vi "On Compile - Cyclic Tx - Get Disable Channels Refs.vi"(8 "error in (no error)":errorcluster, 10 "Channel Data [] In":T1[](array[typedef]) {"Labels Settings"."Label Timestamp Channel Data Reference" format="%.0x"; "Labels Settings"."Label Disable/Trigger Channel Reference" format="%.0x"; "Labels Settings"."Word"."Param Setting"."Item Refs" format="%.0x"; "Labels Settings"."Word"."Param Setting"."Num Bits" min=1 max=32; "Labels Settings"."Word"."Param Setting"."Start Bit" min=8 max=31; "Labels Settings"."Label" format="%.0o"}) -> (0 "error out":errorcluster, 3 "Async Status Channels Refs":T13 {"VS Refs" format="%.0x"})   [LabVIEW 2019, in "Ballard Arinc-429 System Explorer.lvlib"]
uses:
  Ballard Arinc-429 System Explorer.lvlib
  <vilib>/NI VeriStand/Custom Device API/Custom Device Item Ref.ctl
  Shared/Controls and Global/RT HW Channel.ctl
  Shared/Controls and Global/RT Label Settings.ctl
  Shared/Controls and Global/Label.ctl
  Shared/Controls and Global/transferPeriod.ctl
  Shared/Controls and Global/RT Word Settings.ctl
  Shared/Controls and Global/RT Param Setting.ctl
  Shared/Controls and Global/Start Bit.ctl
  Shared/Controls and Global/Number of Bits.ctl
  <vilib>/NI VeriStand/Custom Device API/Block Data Reference.ctl
  <vilib>/NI VeriStand/Custom Device API/Data Reference.ctl
  Shared/Controls and Global/TransferType.ctl
  <vilib>/NI VeriStand/Custom Device API/Custom Device API.lvlib
  Shared/Ballard Arinc-429 Shared.lvlib
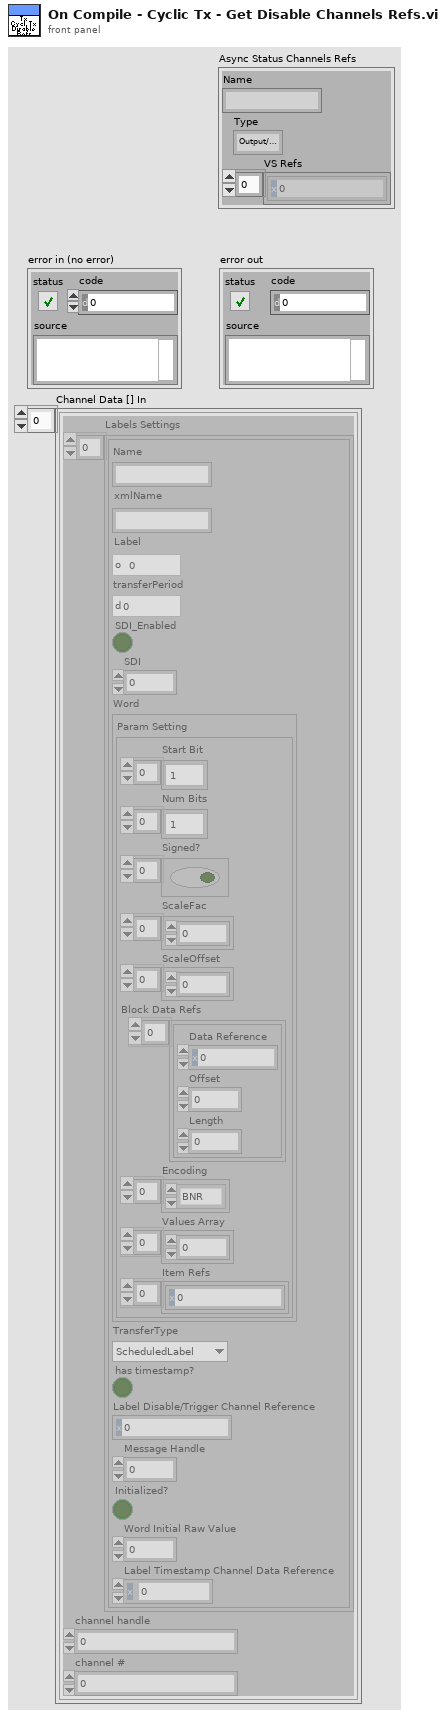
[diagram p1: front panel]
types:
  T1 = typedef "Ballard Arinc-429 Shared.lvlib/RT HW Channel.ctl" = cluster{"Labels Settings":T2[], "channel handle":u64, "channel #":u16}
  T2 = typedef "Ballard Arinc-429 Shared.lvlib/RT Label Settings.ctl" = cluster{"Name":string, "xmlName":string, "Label":T3, "transferPeriod":T4, "SDI_Enabled":bool, "SDI":u8, "Word":T5, "TransferType":T12, "has timestamp?":bool, "Label Disable/Trigger Channel Reference":T11, "Message Handle":u64, "Initialized?":bool, "Word Initial Raw Value":u32, "Label Timestamp Channel Data Reference":T10}
  T3 = typedef "Ballard Arinc-429 Shared.lvlib/Label.ctl" = u8
  T4 = typedef "Ballard Arinc-429 Shared.lvlib/transferPeriod.ctl" = u32
  T5 = typedef "Ballard Arinc-429 Shared.lvlib/RT Word Settings.ctl" = cluster{"Param Setting":T6}
  T6 = typedef "Ballard Arinc-429 Shared.lvlib/RT Param Setting.ctl" = cluster{"Start Bit":T7[], "Num Bits":T8[], "Signed?":bool[], "ScaleFac":dbl[], "ScaleOffset":dbl[], "Block Data Refs":T9[], "Encoding":enum16{"BNR", "BCD", "Discrete"}[], "Values Array":dbl[], "Item Refs":T11[]}
  T7 = typedef "Ballard Arinc-429 Shared.lvlib/Start Bit.ctl" = i32
  T8 = typedef "Ballard Arinc-429 Shared.lvlib/Number of Bits.ctl" = i32
  T9 = typedef "Custom Device API.lvlib/Block Data Reference.ctl" = cluster{"Data Reference":T10, "Offset":u64, "Length":u64}
  T10 = typedef "Custom Device API.lvlib/Data Reference.ctl" = i32
  T11 = typedef "Custom Device API.lvlib/Custom Device Item Ref.ctl" = u64
  T12 = typedef "Ballard Arinc-429 Shared.lvlib/TransferType.ctl" = enum16{"ScheduledLabel", "Acyclic", "Block", "Strobe"}
  T13 = cluster{"Name":string, "Type":enum16{"Output/Write", "Input/Read", "Input/ReadWrite"}, "VS Refs":T11[]}
  T14 = enum16{"Output/Write", "Input/Read", "Input/ReadWrite"}
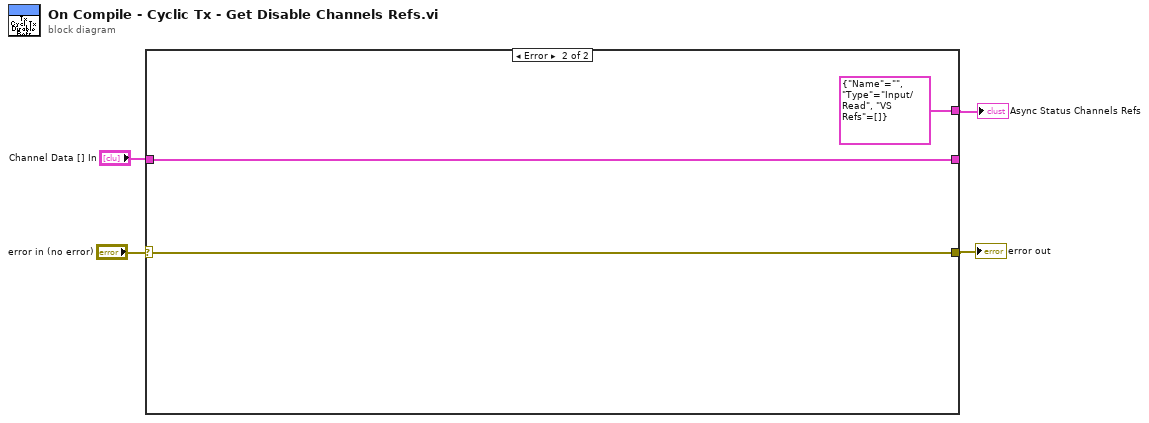
[diagram p0: block diagram]
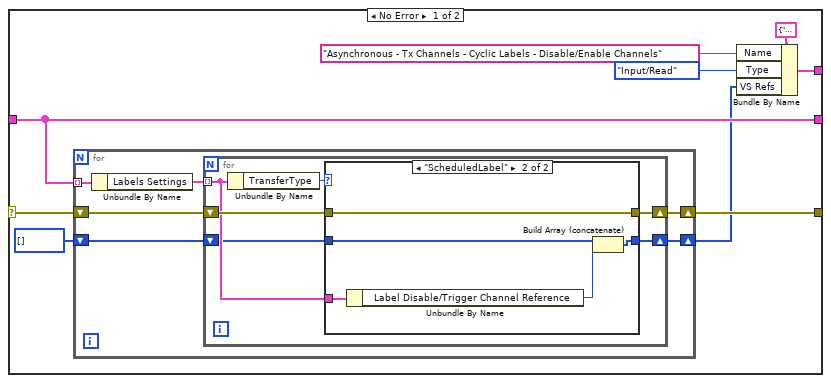
[diagram p2: hidden frame]
diagram:
  n1 = case shown="Error" "error in (no error)" {
    selector: "error in (no error)" -> [w13 w35]
    tunnel: [w11 w35] -> w3
    tunnel: "Channel Data [] In" -> [w12 w34]
    tunnel: [w12 w34] -> _
    tunnel: [w7 T13 {"Name"="", "Type"=enum."Input/Read", "VS Refs"=[]} ("Group")] -> w1
    frame No Error {
      n2 = for {
        tunnel: w12 -> [w19] mode=indexing
        shift-right: [w16] -> w11
        shift-left: w13 -> [w18]
        shift-right: [w15] -> w8
        shift-left: T11[] [] -> [w14]
        n3 = Unbundle By Name(w19) -> ("Labels Settings"=w17:T2[])
        n4 = for {
          shift-right: [w23] -> w16
          shift-left: w18 -> [w24]
          tunnel: w17 -> [w22] mode=indexing
          shift-right: [w21] -> w15
          shift-left: w14 -> [w20]
          n5 = Unbundle By Name(w22) -> ("TransferType"=w25:T12)
          n6 = case shown="\"ScheduledLabel\"" w25 {
            tunnel: w24 -> [w27 w28]
            tunnel: [w27 w28] -> w23
            tunnel: w22 -> [_ w32]
            tunnel: [w26 w30] -> w21
            tunnel: w20 -> [w26 w29]
            frame "Acyclic", Default {
            }
            frame "ScheduledLabel" {
              n7 = Unbundle By Name(w32) -> ("Label Disable/Trigger Channel Reference"=w31:T11)
              n8 = Build Array (concatenate)(w29, w31) -> (w30:T11[])
            }
          }
        }
      }
      n9 = Bundle By Name(cluster=T13 {"Name"="", "Type"=enum."Output/Write", "VS Refs"=[]} ("Group"), "Name"="Asynchronous - Tx Channels - Cyclic Labels - Disable/Enable Channels", "Type"=T14."Input/Read", "VS Refs"=w8) -> (w7:T13)
    }
    frame Error {
    }
  }
  "error out" <- w3
  "Async Status Channels Refs" <- w1
